vi "Template Library Path.vi"() -> (2 "Template Library Path":path)   [LabVIEW 2020, in "LV-Protoc.lvlib"]
uses:
  LV-Protoc.lvlib
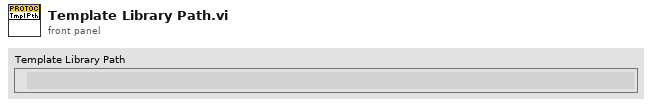
[diagram p1: front panel]
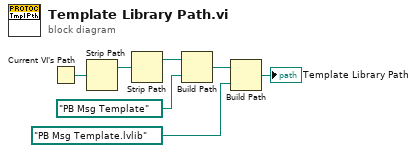
[diagram p0: block diagram]
diagram:
  n1 = Current VI's Path() -> (path=w7:path)
  n2 = Strip Path(path=w7) -> (stripped path=w6:path)  [unwired: 1 out]
  n3 = Strip Path(path=w6) -> (stripped path=w5:path)  [unwired: 1 out]
  n4 = Build Path(base path=w5, name or relative path=path "PB Msg Template") -> (appended path=w3:path)
  n5 = Build Path(base path=w3, name or relative path=path "PB Msg Template.lvlib") -> (appended path=→"Template Library Path":path)
